vi "timeelapsed.vi"() -> (0 "validity":bool, 1 "dt":u32)   [LabVIEW 2017]
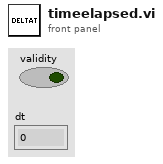
[diagram p1: front panel]
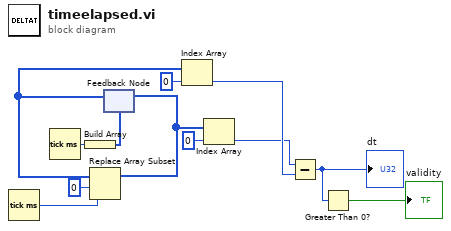
[diagram p0: block diagram]
diagram:
  n1 = Tick Count (ms)() -> (millisecond timer value=w3:u32)
  n2 = Tick Count (ms)() -> (millisecond timer value=w1:u32)
  n3 = Build Array(w1) -> (w2:u32[])
  n4 = feedback #1(w2) -> (w5:u32[])
  n5 = Replace Array Subset(array=w5, new element=w3, index=0) -> (w4:u32[])
  n6 = feedback-in #1(w4) -> ()
  n7 = Index Array(array=w5, index=0) -> (element=w10:u32)
  n8 = Index Array(array=w4, index=0) -> (element=w9:u32)
  n9 = Subtract(x=w9, y=w10) -> (x-y=w11:u32)
  "dt" <- w11
  n10 = Greater Than 0?(x=w11) -> (x > 0?=→"validity":bool)
